vi "csv-db.vi"(7 "db path":path, 8 "error in (no errror)":errorcluster, 11 "results path":path) -> (0 "error out":errorcluster)   [LabVIEW 2024]
uses:
  <vilib>/drjdpowell/SQLite Library/SQL Connection/Open (path).vi
  <vilib>/drjdpowell/SQLite Library/SQL Connection/Open (string).vi
  <vilib>/Utility/file.llb/Read Delimited Spreadsheet (string).vi
  <vilib>/AdvancedString/Path To Command Line String.vi
  <vilib>/drjdpowell/SQLite Library/SQL Connection/Execute SQL (Single Integer).vi
  <vilib>/drjdpowell/SQLite Library/SQL Connection/Execute SQL (No results).vi
  <vilib>/drjdpowell/SQLite Library/SQL Connection/Connection.lvclass
  <vilib>/drjdpowell/SQLite Library/SQLite.lvlib
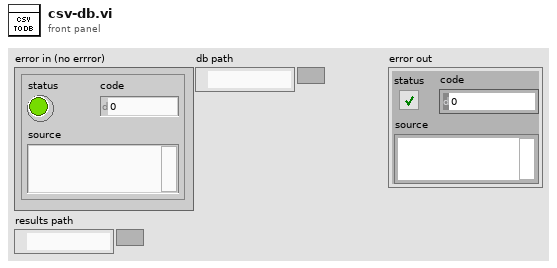
[diagram p1: front panel]
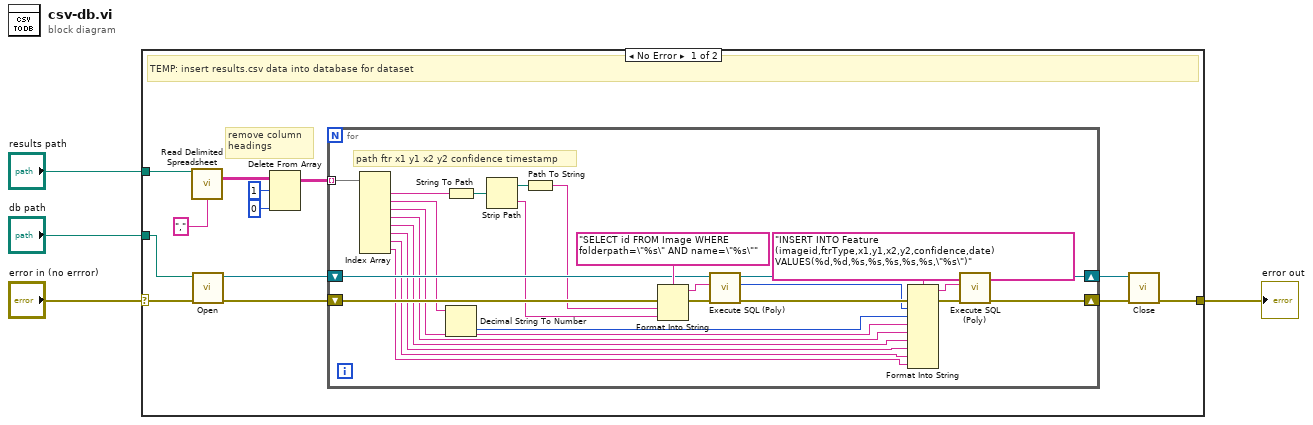
[diagram p0: block diagram]
diagram:
  n1 = case shown="No Error" "error in (no errror)" {
    selector: "error in (no errror)" -> [w17 w45]
    tunnel: [w15 w45] -> w3
    tunnel: "results path" -> [w10 _]
    tunnel: "db path" -> [w13 _]
    frame No Error {
      # "remove column\nheadings"
      # "TEMP: insert results.csv data into database for dataset"
      n2 = call-poly <vilib>:"Read Delimited Spreadsheet.vi"("file path (dialog if empty)"=w10, "delimiter (\\t)"="," ("delimiter (\\t)")) -> ("all rows"=w9:string[][])  [unwired: 8 in, 5 out]
      n3 = call-poly <vilib>:"Open.vi"("error in (no error)"=w17, "db file"=w13) -> ("error out"=w12:errorcluster, "SQLite Connection"=w11:refnum<class "Connection.lvclass">)  [unwired: 8 in]
      n4 = Delete From Array(array=w9, length=1, index (row)=0) -> (array with subset deleted=w6:string[][])  [unwired: 1 in, 1 out]
      n5 = for {
        shift-right: [w44] -> w16
        shift-left: w12 -> [w38]
        shift-right: [w43] -> w14
        shift-left: w11 -> [w35]
        tunnel: w6 -> [w33] mode=indexing
        # "path ftr x1 y1 x2 y2 confidence timestamp"
        n6 = Index Array(array=w33) -> (element #1=w31:string, element #2=w19:string, element #3=w26:string, element #4=w25:string, element #5=w24:string, element #6=w23:string, element #7=w22:string, element #8=w21:string)  [unwired: 8 in]
        n7 = String To Path(string=w31) -> (path=w30:path)
        n8 = Decimal String To Number(string=w19) -> (number=w18:i32)  [unwired: 2 in, 1 out]
        n9 = Strip Path(path=w30) -> (stripped path=w28:path, name=w29:string)
        n10 = Path To String(path=w28) -> (string=w27:string)
        n11 = Format Into String(format string="SELECT id FROM Image WHERE folderpath=\"%s\" AND name=\"%s\"", error in=w38, w27, w29) -> (resulting string=w32:string, error out=w39:errorcluster)  [unwired: 1 in]
        n12 = call-poly <vilib>:"Execute SQL (Poly).vi"("error in (no error)"=w39, "SQL"=w32, "SQLite Connection in"=w35) -> ("error out"=w36:errorcluster, "Result"=w20:i64, "SQLite Connection"=w34:refnum<class "Connection.lvclass">)  [unwired: 6 in]
        n13 = Format Into String(format string="INSERT INTO Feature (imageid,ftrType,x1,y1,x2,y2,confidence,date) VALUES(%d,%d,%s,%s,%s,%s,%s,\"%s\")", error in=w36, w20, w18, w26, w25, w24, w23, w22, w21) -> (resulting string=w41:string, error out=w42:errorcluster)  [unwired: 1 in]
        n14 = call-poly <vilib>:"Execute SQL (Poly).vi"("error in (no error)"=w42, "SQL"=w41, "SQLite Connection in"=w34) -> ("error out"=w44:errorcluster, "SQLite Connection"=w43:refnum<class "Connection.lvclass">)  [unwired: 7 in]
      }
      n15 = call-dynamic "Close.vi"("error in (no error)"=w16, "SQLite Connection in"=w14) -> ("error out"=w15:errorcluster)  [unwired: 9 in]
    }
    frame Error {
    }
  }
  "error out" <- w3
